vi "VISA terminate.vi"(8 "error in (no error)":errorcluster, 11 "AOTF in":refnum<class "AOTF.lvclass">) -> (0 "error out":errorcluster, 3 "AOTF out":refnum<class "AOTF.lvclass">)   [LabVIEW 2012, in "AOTF.lvclass"]
uses:
  AOTF.lvclass
  AOTF.lvclass/AOTF.ctl
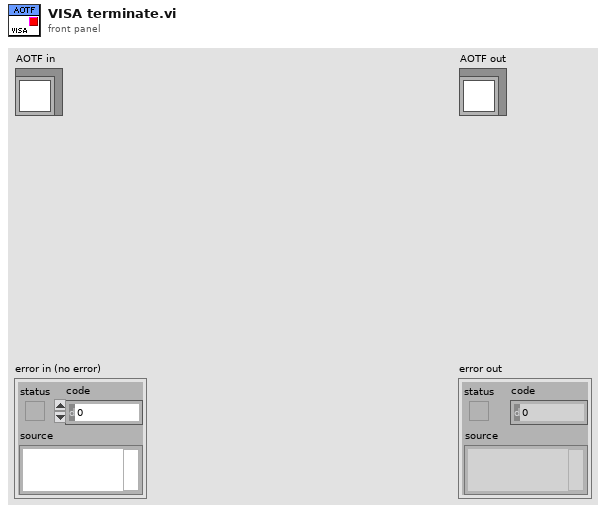
[diagram p1: front panel]
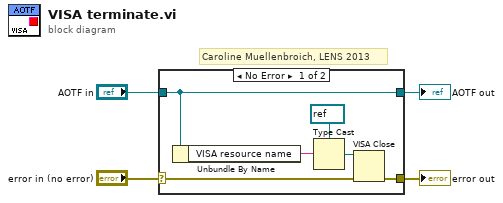
[diagram p0: block diagram]
diagram:
  # "Caroline Muellenbroich, LENS 2013"
  n1 = case shown="No Error" "error in (no error)" {
    selector: "error in (no error)" -> [w10 w12]
    tunnel: [w9 w12] -> w3
    tunnel: [w8 w11] -> w1
    tunnel: "AOTF in" -> [w8 w11]
    frame No Error {
      n2 = Unbundle By Name(w8) -> ("VISA resource name"=w7:string)
      n3 = Type Cast(type=refnum<visa-resource-name> refnum ("VISA resource name"), x=w7) -> (*(type *) &x=w5:refnum<visa-resource-name>)
      n4 = VISA Close(VISA resource name=w5, error in (no error)=w10) -> (error out=w9:errorcluster)
    }
    frame Error {
    }
  }
  "error out" <- w3
  "AOTF out" <- w1
